vi "LJU3_temp_status.vi"(4 "lolo":dbl=85.0, 5 "hihi":dbl=115.0, 6 "lo":dbl=90.0, 7 "hi":dbl=110.0, 9 "T":dbl[](array[numeric]) format="%.1f", 11 "readout_status":bool) -> (1 "temp_status":T1)   [LabVIEW 2019]
uses:
  temperature_status_LabJackU3.ctl
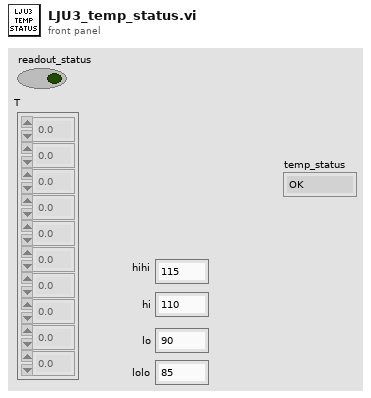
[diagram p1: front panel]
types:
  T1 = typedef "temperature_status_LabJackU3.ctl" = enum16{"OK", "UNKNOWN", "WARNING", "ERROR"}
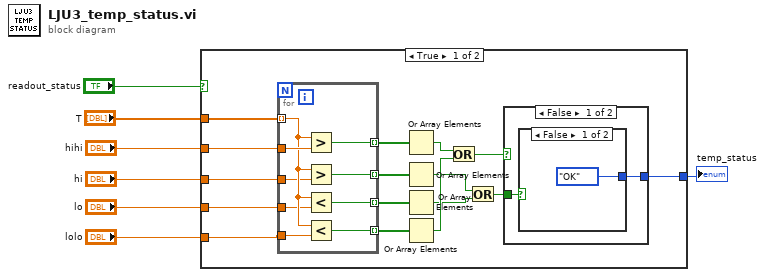
[diagram p0: block diagram]
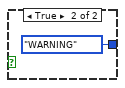
[diagram p2: hidden frame]
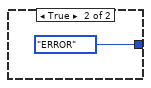
[diagram p3: hidden frame]
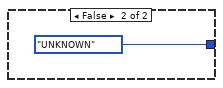
[diagram p4: hidden frame]
diagram:
  n1 = case shown="True" "readout_status" {
    tunnel: "T" -> [w23 _]
    tunnel: "hihi" -> [w22 _]
    tunnel: "hi" -> [w20 _]
    tunnel: "lo" -> [w19 _]
    tunnel: "lolo" -> [w18 _]
    tunnel: [w8 temperature_status_LabJackU3."UNKNOWN" ("temp_status")] -> w1
    frame True {
      n2 = for {
        tunnel: w23 -> [w35] mode=indexing
        tunnel: w22 -> [w37]
        tunnel: [w36] -> w21 mode=indexing
        tunnel: w20 -> [w34]
        tunnel: w19 -> [w33]
        tunnel: w18 -> [w32]
        tunnel: [w31] -> w17 mode=indexing
        tunnel: [w30] -> w16 mode=indexing
        tunnel: [w29] -> w15 mode=indexing
        n3 = Greater?(x=w35, y=w37) -> (0:w36:bool)
        n4 = Greater?(x=w35, y=w34) -> (0:w31:bool)
        n5 = Less?(x=w35, y=w33) -> (x < y?=w30:bool)
        n6 = Less?(x=w35, y=w32) -> (x < y?=w29:bool)
      }
      n7 = Or Array Elements(Boolean array=w21) -> (logical OR=w14:bool)
      n8 = Or Array Elements(Boolean array=w17) -> (logical OR=w12:bool)
      n9 = Or Array Elements(Boolean array=w16) -> (logical OR=w11:bool)
      n10 = Or Array Elements(Boolean array=w15) -> (logical OR=w13:bool)
      n11 = Or(x=w14, y=w13) -> (x .or. y?=w10:bool)
      n12 = Or(x=w12, y=w11) -> (x .or. y?=w9:bool)
      n13 = case shown="False" w10 {
        tunnel: w9 -> [w25 _]
        tunnel: [w24 temperature_status_LabJackU3."ERROR" ("temp_status")] -> w8
        frame False {
          n14 = case shown="False" w25 {
            tunnel: [temperature_status_LabJackU3."OK" ("temp_status") temperature_status_LabJackU3."WARNING" ("temp_status")] -> w24
            frame False {
            }
            frame True {
            }
          }
        }
        frame True {
        }
      }
    }
    frame False {
    }
  }
  "temp_status" <- w1
